vi "Thermometer.vi"(8 "error in (no error)":errorcluster) -> (0 "error out":errorcluster, 2 "Humidity while Roasting":dbl(knob) scale=0.0..100.0 scale format="%.1f")   [LabVIEW 2018]
doc: "This VI simulates measuring a temperature using the temperature sensor on the DAQ Signal Accessory.\n\nIf you have a DAQ board or a DAQ Signal Accessory, then use the Thermometer VI instead."
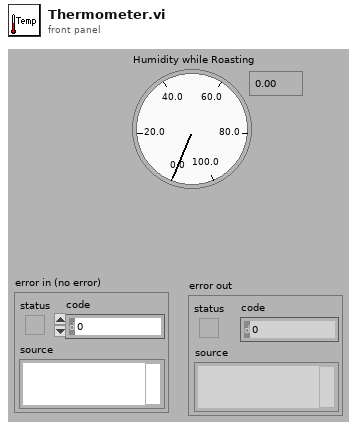
[diagram p1: front panel]
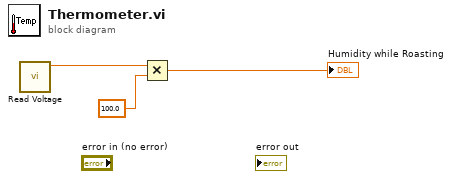
[diagram p0: block diagram]
diagram:
  n1 = call "Read Voltage.vi"() -> ("voltage"=w2:dbl)  [unwired: 1 in, 6 out]
  n2 = Multiply(x=w2, y=100.0) -> (x*y=→"Humidity while Roasting":dbl)
